vi "Package Data.vi"(8 "error in (no error)":errorcluster, 9 "LED Outputs":T2, 10 "PWM Outputs":T1, 11 "VISA resource name in":refnum<visa-resource-name>) -> (0 "error out":errorcluster, 3 "VISA resource name out":refnum<visa-resource-name>)   [LabVIEW 2013]
uses:
  LED_Output_TypeDef.ctl
  PWM_Output_TypeDef.ctl
  CRC SubVIs/Wrappers/CRC-8-Maxim 1-Wire (DOW).vi
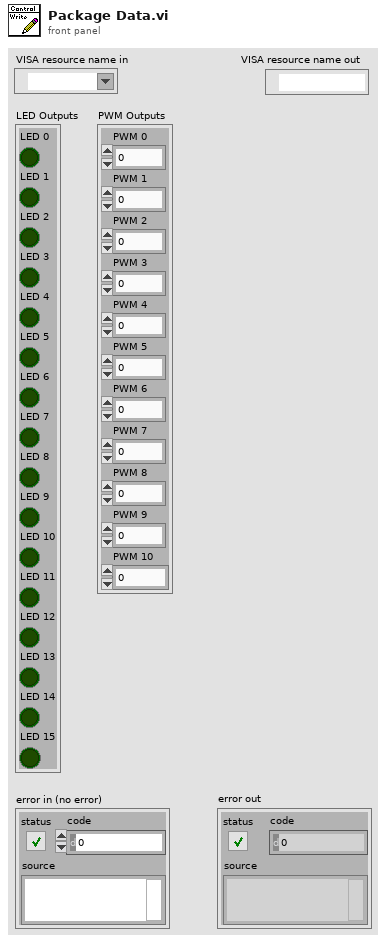
[diagram p1: front panel]
types:
  T1 = typedef "PWM_Output_TypeDef.ctl" = cluster{"PWM 0":u8, "PWM 1":u8, "PWM 2":u8, "PWM 3":u8, "PWM 4":u8, "PWM 5":u8, "PWM 6":u8, "PWM 7":u8, "PWM 8":u8, "PWM 9":u8, "PWM 10":u8}
  T2 = typedef "LED_Output_TypeDef.ctl" = cluster{"LED 0":bool, "LED 1":bool, "LED 2":bool, "LED 3":bool, "LED 4":bool, "LED 5":bool, "LED 6":bool, "LED 7":bool, "LED 8":bool, "LED 9":bool, "LED 10":bool, "LED 11":bool, "LED 12":bool, "LED 13":bool, "LED 14":bool, "LED 15":bool}
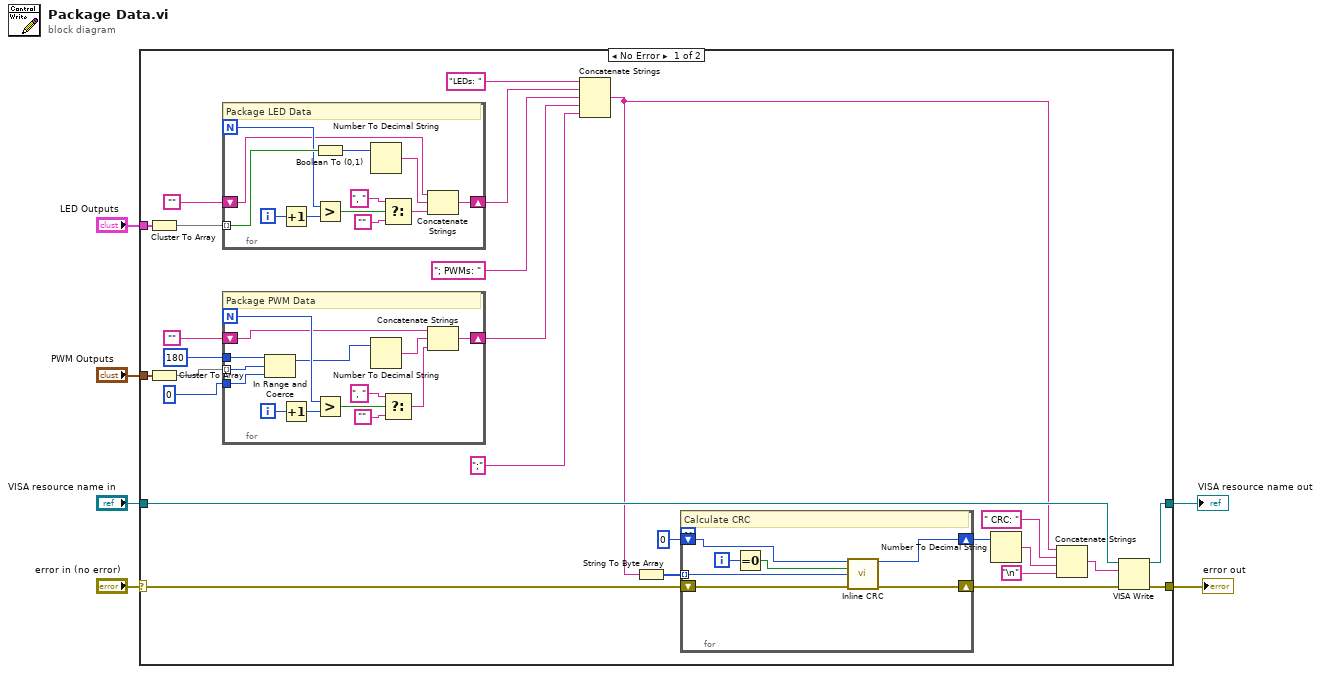
[diagram p0: block diagram]
diagram:
  n1 = case shown="No Error" "error in (no error)" {
    selector: "error in (no error)" -> [w7 w67]
    tunnel: "LED Outputs" -> [w17 _]
    tunnel: "PWM Outputs" -> [w16 _]
    tunnel: [w14 w67] -> w4
    tunnel: "VISA resource name in" -> [w13 w66]
    tunnel: [w12 w66] -> w2
    frame No Error {
      n2 = Cluster To Array(cluster=w17) -> (array=w18:bool[])
      n3 = Cluster To Array(cluster=w16) -> (array=w20:u8[])
      n4 = for {
        N -> [w62]
        tunnel: w18 -> [w65] mode=indexing
        shift-right: [w56] -> w25
        shift-left: "" -> [w57]
        i -> [w60]
        # "Package LED Data"
        n5 = Increment(x=w60) -> (x+1=w61:i32)
        n6 = Boolean To (0,1)(Boolean=w65) -> (0, 1=w64:i16)
        n7 = Greater?(x=w62, y=w61) -> (0:w59:bool)
        n8 = Number To Decimal String(number=w64) -> (decimal integer string=w63:string)  [unwired: 1 in]
        n9 = Select(t=", ", s=w59, f="") -> (s? t:f=w58:string)
        n10 = Concatenate Strings(w57, w63, w58) -> (w56:string)
      }
      n11 = for {
        N -> [w52]
        tunnel: w20 -> [w43] mode=indexing
        shift-right: [w46] -> w27
        shift-left: "" -> [w47]
        tunnel: u8 0 ("upper limit") -> [w41]
        tunnel: u8 180 ("upper limit") -> [w40]
        i -> [w50]
        # "Package PWM Data"
        n12 = In Range and Coerce(upper limit=w40, x=w43, lower limit=w41) -> (coerced(x)=w42:u8)  [unwired: 1 out]
        n13 = Increment(x=w50) -> (x+1=w51:i32)
        n14 = Greater?(x=w52, y=w51) -> (0:w49:bool)
        n15 = Number To Decimal String(number=w42) -> (decimal integer string=w53:string)  [unwired: 1 in]
        n16 = Select(t=", ", s=w49, f="") -> (s? t:f=w48:string)
        n17 = Concatenate Strings(w47, w53, w48) -> (w46:string)
      }
      n18 = Concatenate Strings("LEDs: " ("string"), w25, "; PWMs: " ("string"), w27, ";" ("string")) -> (w10:string)
      n19 = String To Byte Array(string=w10) -> (unsigned byte array=w28:u8[])
      n20 = for {
        tunnel: w28 -> [w39] mode=indexing
        shift-right: [w37] -> w30
        shift-left: u8 0 ("CRC In") -> [w38]
        shift-right: [w35] -> w15
        shift-left: w7 -> [w36]
        i -> [w34]
        # "Calculate CRC"
        n21 = Equal To 0?(x=w34) -> (x = 0?=w33:bool)
        n22 = call-poly "Inline CRC.vi"("CRC In"=w38, "Reset"=w33, "Data"=w39, "error in (no error)"=w36) -> ("CRC"=w37:u8, "error out"=w35:errorcluster)  [unwired: 10 in]
      }
      n23 = Number To Decimal String(number=w30) -> (decimal integer string=w31:string)  [unwired: 1 in]
      n24 = Concatenate Strings(w10, " CRC: " ("string"), w31, "\n") -> (w8:string)
      n25 = VISA Write(VISA resource name=w13, write buffer=w8, error in (no error)=w15) -> (VISA resource name out=w12:refnum<visa-resource-name>, error out=w14:errorcluster)  [unwired: 1 out]
    }
    frame Error {
    }
  }
  "error out" <- w4
  "VISA resource name out" <- w2
